vi "Timer Running Control.vi"(11 "Enum":T1(ring)) -> (3 "Timer State":bool)   [LabVIEW 2013]
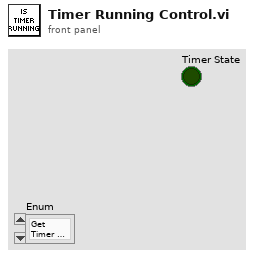
[diagram p1: front panel]
types:
  T1 = enum16{"Get Timer State", "Start Timer", "Stop Timer"}
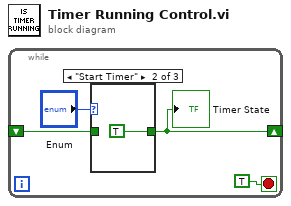
[diagram p0: block diagram]
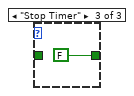
[diagram p3: hidden frame]
diagram:
  n1 = while {
    shift-right: [w2] -> _
    shift-left: _ -> [w1]
    stop <- TRUE stop-if-true
    n2 = case shown="\"Start Timer\"" "Enum" {
      tunnel: [w5 TRUE FALSE] -> w2
      tunnel: w1 -> [w5 _ _]
      frame "Get Timer State", Default {
      }
      frame "Start Timer" {
      }
      frame "Stop Timer" {
      }
    }
    "Timer State" <- w2
  }
